vi "Create Waveform and Preview.vi"(5 "XYGraph Refnum":refnum<vi>, 7 "Program":T3(array[cluster]), 8 "error in (no error)":errorcluster, 10 "Waveform In":T1, 11 "Display State In":T2 caption="State" {"# of Loops" min=1 step=1; "Index" min=0 step=1; "Program"."Step" min=0.001 max=80.0 step=0.001 format="%.2f"; "Program"."Target" format="%.2f"}) -> (0 "error out":errorcluster, 1 "Preview Graph":cluster{dbl[], dbl[]}[](graph), 2 "Waveform Out":T1, 3 "State Out":T2 caption="State" {"# of Loops" min=1 step=1; "Index" min=0 step=1; "Program"."Step" min=0.001 max=80.0 step=0.001 format="%.2f"; "Program"."Target" format="%.2f"})   [LabVIEW 2012, in "Multi Segment Waveform.xctl"]
doc: "Build Preview with current marker and y=0 line"
uses:
  Multi Segment Waveform.xctl
  State.ctl
  Data.ctl
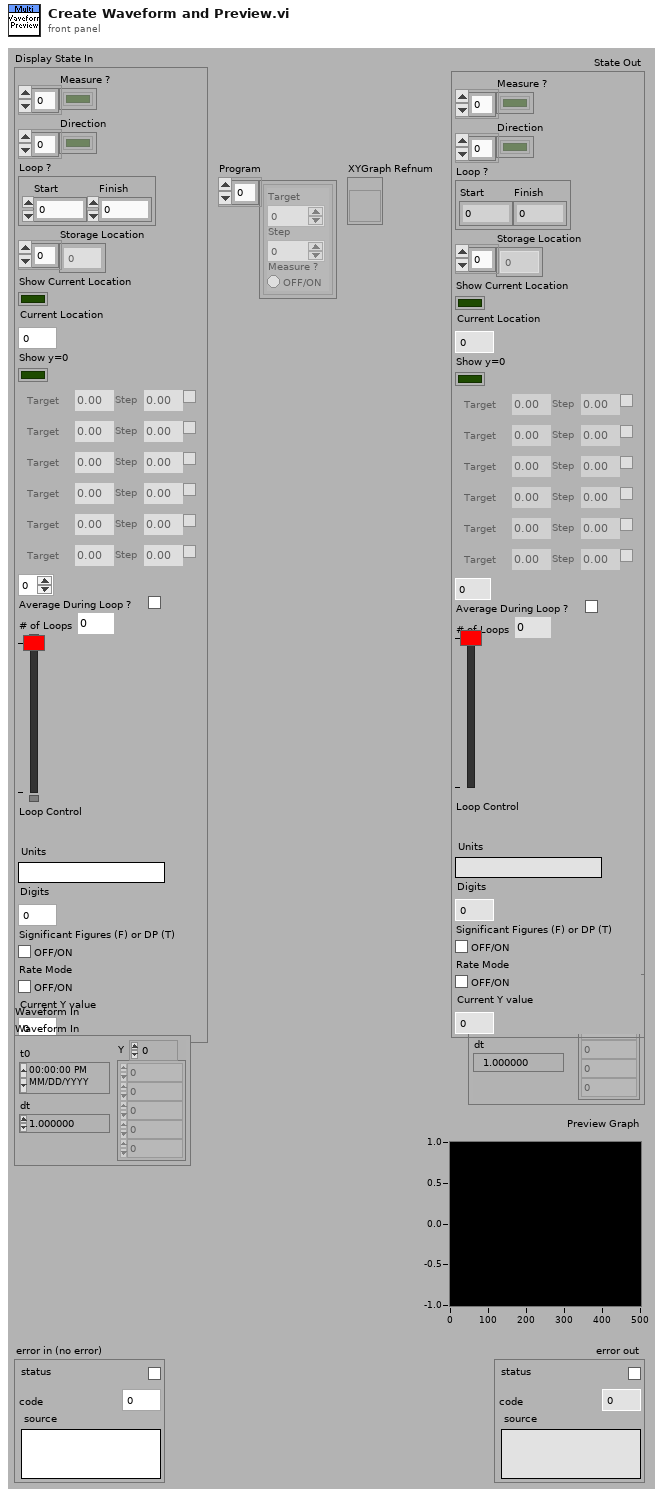
[diagram p1: front panel]
types:
  T1 = typedef "Multi Segment Waveform.xctl/Data.ctl" = waveform(dbl)
  T2 = typedef "Multi Segment Waveform.xctl/State.ctl" = cluster{"Measure ?":bool[], "Direction":bool[], "Loop ?":cluster{"Start":i32, "Finish":i32}, "Storage Location":i32[], "Show Current Location":bool, "Current Location":i32, "Show y=0":bool, "Program":cluster{"Target":dbl, "Step":dbl, "Measure ?":bool}[], "Index":i32, "Average During Loop ?":bool, "# of Loops":u32, "Loop Control":cluster{i32, i32}, "Units":string, "Digits":i32, "Significant Figures (F) or DP (T)":bool, "Rate Mode":bool, "Current Y value":dbl}
  T3 = cluster{"Target":dbl, "Step":dbl, "Measure ?":bool}[]
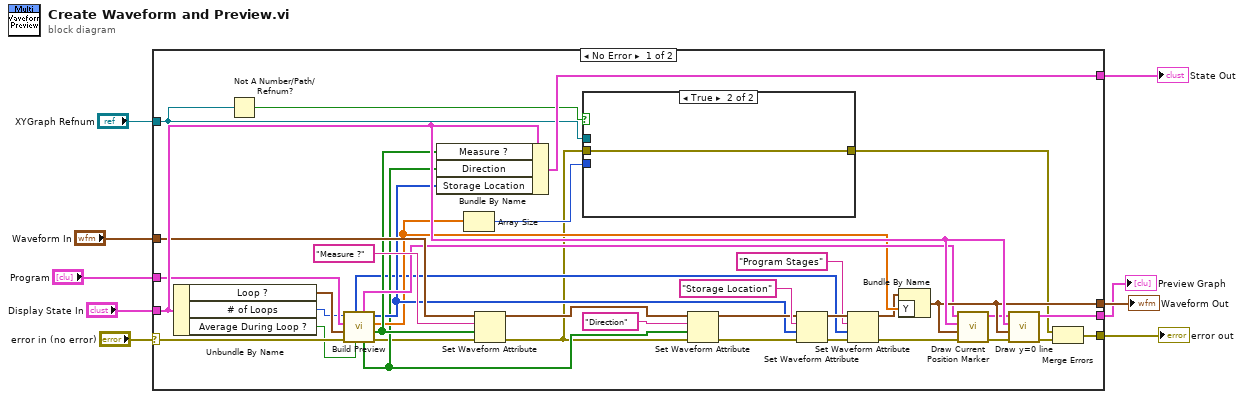
[diagram p0: block diagram]
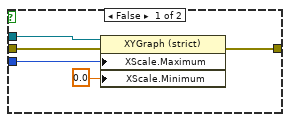
[diagram p2: hidden frame]
diagram:
  n1 = case shown="No Error" "error in (no error)" {
    selector: "error in (no error)" -> [w24 w54]
    tunnel: "Display State In" -> [w46 w53]
    tunnel: [w44 _] -> w8
    tunnel: [w43 _] -> w7
    tunnel: "Program" -> [w36 _]
    tunnel: [w35 w53] -> w5
    tunnel: "Waveform In" -> [w34 _]
    tunnel: "XYGraph Refnum" -> [w14 _]
    tunnel: [w12 w54] -> w1
    frame No Error {
      n2 = Unbundle By Name(w46) -> ("Loop ?"=w33:cluster{"Start":i32, "Finish":i32}, "# of Loops"=w16:u32, "Average During Loop ?"=w15:bool)
      n3 = Not A Number/Path/Refnum?(number/path/refnum=w14) -> (NaN/Path/Refnum?=w10:bool)
      n4 = call "Build Preview.vi"("Average During Loop ?"=w15, "error in (no error)"=w24, "Loop ?"=w33, "Program"=w36, "# Of Loops"=w16) -> ("error out"=w25:errorcluster, "Measure ? Out"=w31:bool[], "Y Values Out"=w29:dbl[], "Storage Locations Out"=w30:i32[], "Direction Out"=w26:bool[], "Plots Out"=w32:cluster{dbl[], dbl[]}[], "Stage Values"=w20:i32[])
      n5 = Bundle By Name(cluster=w46, "Measure ?"=w31, "Direction"=w26, "Storage Location"=w30) -> (w35:T2)
      n6 = Array Size(array=w29) -> (size(s)=w45:i32)
      n7 = Set Waveform Attribute(4:w25, 5:w31, 6:"Measure ?" ("name"), 7:w34) -> (0:w13:errorcluster, 3:w37:T1)  [unwired: 1 out]
      n8 = case shown="True" w10 {
        tunnel: w45 -> [w50 _]
        tunnel: w14 -> [w49 _]
        tunnel: w13 -> [w48 w52]
        tunnel: [w47 w52] -> w11
        frame False {
          n9 = property on="Property Node" class="XYGraph (strict)"(reference=w49, error in=w48, "XScale.Maximum"=w50, "XScale.Minimum"=0.0 ("X Scale.Range:Minimum")) -> (error out=w47:errorcluster)  [unwired: 1 out]
        }
        frame True {
        }
      }
      n10 = Set Waveform Attribute(4:w13, 5:w26, 6:"Direction" ("name"), 7:w37) -> (0:w27:errorcluster, 3:w38:T1)  [unwired: 1 out]
      n11 = Set Waveform Attribute(4:w27, 5:w30, 6:"Storage Location" ("name"), 7:w38) -> (0:w22:errorcluster, 3:w21:T1)  [unwired: 1 out]
      n12 = Set Waveform Attribute(4:w22, 5:w20, 6:"Program Stages" ("name"), 7:w21) -> (0:w17:errorcluster, 3:w18:T1)  [unwired: 1 out]
      n13 = Bundle By Name(cluster=w18, "Y"=w29) -> (w44:T1)
      n14 = call "Draw Current Position Marker.vi"("Error"=w17, "Waveform"=w44, "State"=w46, "Plots"=w32) -> ("Error Out"=w28:errorcluster, "Plots Out"=w42:cluster{"X":dbl[], "Y":dbl[]}[])  [unwired: 6 out]
      n15 = call "Draw y=0 line.vi"("Error"=w28, "Waveform"=w44, "State"=w46, "Plots"=w42) -> ("Error Out"=w23:errorcluster, "Plots Out"=w43:cluster{"X":dbl[], "Y":dbl[]}[])  [unwired: 6 out]
      n16 = Merge Errors(w11, w23) -> (w12:errorcluster)
    }
    frame Error {
    }
  }
  "Preview Graph" <- w7
  "Waveform Out" <- w8
  "State Out" <- w5
  "error out" <- w1
